vi "Array To List.vi"(11 "Array":string[](array[string])) -> (3 "String":string)   [LabVIEW 2017, in "LVJSON.lvlib"]
uses:
  LVJSON.lvlib
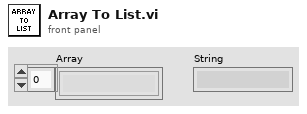
[diagram p1: front panel]
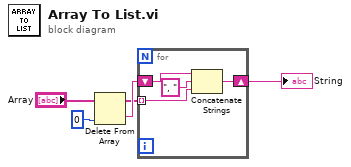
[diagram p0: block diagram]
diagram:
  n1 = Delete From Array(array="Array", index=0) -> (deleted portion=w4:string, array with subset deleted=w3:string[])  [unwired: 1 in]
  n2 = for {
    tunnel: w3 -> [w7] mode=indexing
    shift-right: [w6] -> w5
    shift-left: w4 -> [w9]
    n3 = Concatenate Strings(w9, ", " ("string"), w7) -> (w6:string)
  }
  "String" <- w5
